vi "CPU Load Benchmark.vi"(8 "error in (no error)":errorcluster, 11 "SV B-M (Target) in":refnum<class "SV B-M (Target).lvclass">) -> (0 "error out":errorcluster, 3 "SV B-M (Target) out":refnum<class "SV B-M (Target).lvclass">)   [LabVIEW 2015, in "SV B-M (Target).lvclass"]
uses:
  SV B-M (Target).lvclass
  SV B-M (Target).lvclass/SV B-M (Target).ctl
  <vilib>/Analysis/baseanly.llb/Mean (DBL).vi
  <vilib>/nisyscfg/Close (Hardware).vi
  <vilib>/nisyscfg/Close (System).vi
  Command & Ack - Send Ack.vi
  <vilib>/nisyscfg/nisyscfg.lvlib
  <resource>/objmgr/nisysapi.rc
  <vilib>/Analysis/NI_AALBase.lvlib
panel:
  out "SV Data":variant[][](array[variant])
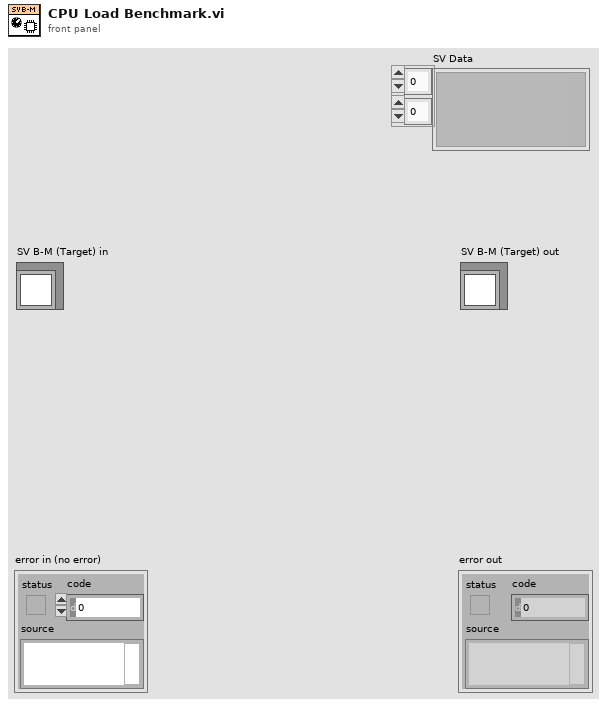
[diagram p1: front panel]
types:
  T1 = typedef "Variable Data Type.ctl" = enum16{"U8", "U16", "U32", "U64", "I8", "I16", "I32", "I64", "Single", "Double", "Boolean", "String"}
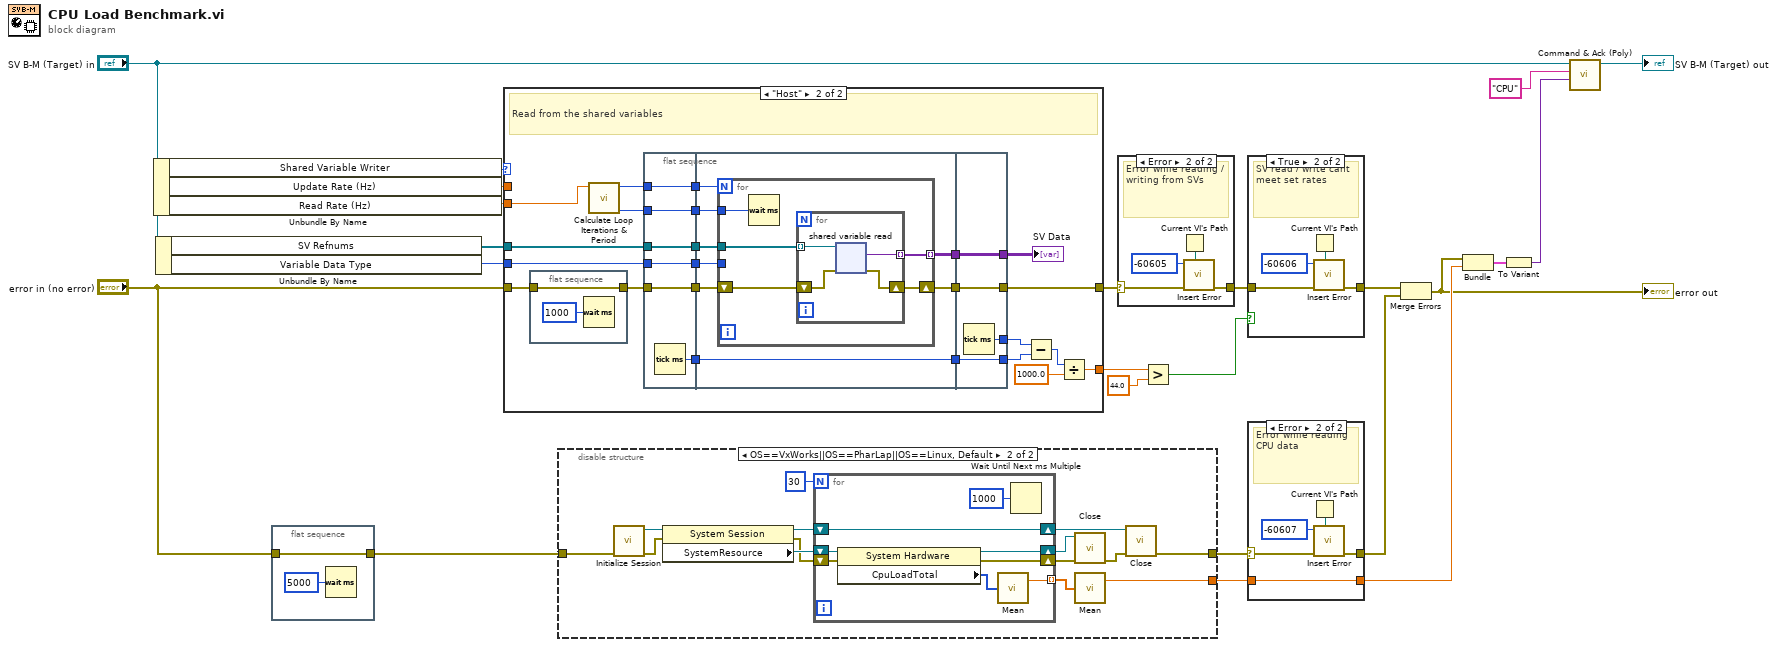
[diagram p0: block diagram]
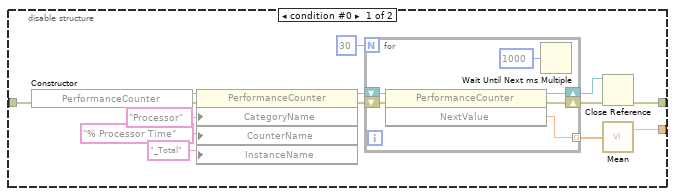
[diagram p3: hidden frame]
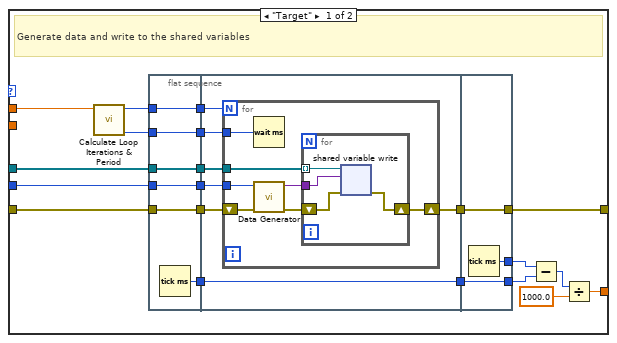
[diagram p6: hidden frame]
diagram:
  n1 = Unbundle By Name("SV B-M (Target) in") -> ("Shared Variable Writer"=w23:enum16{"Target", "Host"}, "Update Rate (Hz)"=w22:dbl, "Read Rate (Hz)"=w21:dbl)
  n2 = Unbundle By Name("SV B-M (Target) in") -> ("SV Refnums"=w20:refnum<k21>[], "Variable Data Type"=w19:T1)
  n3 = flat-sequence {
    tunnel: "error in (no error)" -> [w25]
    tunnel: [w25] -> w12
    frame #0 {
      n4 = Wait (ms)(milliseconds to wait=u32 5000) -> ()  [unwired: 1 out]
    }
  }
  n5 = case shown="\"Host\"" w23 {
    tunnel: w22 -> [w45 _]
    tunnel: w21 -> [_ w78]
    tunnel: w20 -> [w42 w93]
    tunnel: w19 -> [w41 w92]
    tunnel: "error in (no error)" -> [w36 w74]
    tunnel: [w27 w79] -> w15
    tunnel: [w26 w76] -> w18
    frame "Target" {
      # "Generate data and write to the shared variables"
      n6 = call "Calculate Loop Iterations & Period.vi"("Rate"=w45) -> ("Wait (ms)"=w43:u32, "# Iterations"=w44:i32)  [unwired: 9 in]
      n7 = flat-sequence {
        tunnel: w41 -> [w48]
        tunnel: w42 -> [w49]
        tunnel: w43 -> [w50]
        tunnel: w44 -> [w51]
        tunnel: [w51] -> w40
        tunnel: [w50] -> w39
        tunnel: [w49] -> w38
        tunnel: [w48] -> w37
        tunnel: w36 -> [w47]
        tunnel: [w47] -> w35
        tunnel: [w46] -> w34
        tunnel: w40 -> [w58]
        tunnel: w39 -> [w57]
        tunnel: w38 -> [w56]
        tunnel: w37 -> [w55]
        tunnel: w35 -> [w54]
        tunnel: w34 -> [w53]
        tunnel: [w53] -> w33
        tunnel: [w52] -> w32
        tunnel: [w72] -> w31
        tunnel: w33 -> [w72]
        tunnel: w32 -> [w70]
        tunnel: [w71] -> w30
        tunnel: [w70] -> w26
        frame #0 {
          n8 = Tick Count (ms)() -> (millisecond timer value=w46:u32)
        }
        frame #1 {
          n9 = for {
            N: w58 -> [_]
            tunnel: w57 -> [w65]
            tunnel: w56 -> [w62]
            tunnel: w55 -> [w64]
            shift-right: [w59] -> w52
            shift-left: w54 -> [w63]
            n10 = Wait (ms)(milliseconds to wait=w65) -> ()  [unwired: 1 out]
            n11 = call "Data Generator.vi"("error in (no error)"=w63, "Variable Data Type"=w64) -> ("error out"=w60:errorcluster, "Variant"=w61:variant)  [unwired: 8 in]
            n12 = for {
              tunnel: w62 -> [w69] mode=indexing
              tunnel: w61 -> [w67]
              shift-right: [w66] -> w59
              shift-left: w60 -> [w68]
              n13 = shared-variable-write(w69, w68, w67) -> (w66:errorcluster)  [unwired: 1 out]
            }
          }
        }
        frame #2 {
          n14 = Tick Count (ms)() -> (millisecond timer value=w71:u32)
        }
      }
      n15 = Subtract(x=w30, y=w31) -> (x-y=w29:u32)
      n16 = Divide(x=w29, y=1000.0) -> (x/y=w27:dbl)
    }
    frame "Host" {
      # "Read from the shared variables"
      n17 = flat-sequence {
        tunnel: w74 -> [w97]
        tunnel: [w97] -> w73
        frame #0 {
          n18 = Wait (ms)(milliseconds to wait=u32 1000) -> ()  [unwired: 1 out]
        }
      }
      n19 = call "Calculate Loop Iterations & Period.vi"("Rate"=w78) -> ("Wait (ms)"=w94:u32, "# Iterations"=w95:i32)  [unwired: 9 in]
      n20 = flat-sequence {
        tunnel: w92 -> [w100]
        tunnel: w93 -> [w101]
        tunnel: w94 -> [w102]
        tunnel: w95 -> [w103]
        tunnel: [w103] -> w91
        tunnel: [w102] -> w90
        tunnel: [w101] -> w89
        tunnel: [w100] -> w88
        tunnel: [w98] -> w87
        tunnel: [w99] -> w86
        tunnel: w73 -> [w98]
        tunnel: w91 -> [w111]
        tunnel: w90 -> [w110]
        tunnel: w89 -> [w109]
        tunnel: w88 -> [w108]
        tunnel: w87 -> [w107]
        tunnel: w86 -> [w106]
        tunnel: [w106] -> w85
        tunnel: [w105] -> w84
        tunnel: [w104] -> w77
        tunnel: [w124] -> w83
        tunnel: w85 -> [w124]
        tunnel: w84 -> [w121]
        tunnel: [w123] -> w82
        tunnel: [w122] -> w75
        tunnel: w77 -> [w122]
        tunnel: [w121] -> w76
        frame #0 {
          n21 = Tick Count (ms)() -> (millisecond timer value=w99:u32)
        }
        frame #1 {
          n22 = for {
            N: w111 -> [_]
            tunnel: w110 -> [w116]
            tunnel: w109 -> [w115]
            tunnel: w108 -> [_]
            shift-right: [w114] -> w105
            shift-left: w107 -> [w113]
            tunnel: [w112] -> w104 mode=indexing
            n23 = Wait (ms)(milliseconds to wait=w116) -> ()  [unwired: 1 out]
            n24 = for {
              tunnel: w115 -> [w120] mode=indexing
              shift-right: [w118] -> w114
              shift-left: w113 -> [w119]
              tunnel: [w117] -> w112 mode=indexing
              n25 = shared-variable-read(w120, w119) -> (w118:errorcluster, w117:variant)  [unwired: 2 out]
            }
          }
        }
        frame #2 {
          n26 = Tick Count (ms)() -> (millisecond timer value=w123:u32)
        }
      }
      n27 = Subtract(x=w82, y=w83) -> (x-y=w81:u32)
      n28 = Divide(x=w81, y=1000.0) -> (x/y=w79:dbl)
      "SV Data" <- w75
    }
  }
  n29 = disable-structure shown="OS==VxWorks||OS==PharLap||OS==Linux, Default" {
    disable-tunnel: w12 -> [w130 w158]
    disable-tunnel: [w125 w147] -> w11
    disable-tunnel: [w126 w146] -> w10
    frame condition #0 {
      n30 = constructor class="PerformanceCounter"(error in=w130) -> (reference out=w138:refnum<k24>, error out=w137:errorcluster)  [unwired: 2 in, 1 out]
      n31 = property class="PerformanceCounter"(reference=w138, error in=w137, "CategoryName"="Processor", "CounterName"="% Processor Time", "InstanceName"="_Total") -> (reference out=w136:refnum<k24>, error out=w135:errorcluster)
      n32 = for {
        N: 30 -> [_]
        shift-right: [w141] -> w128
        shift-left: w136 -> [w144]
        shift-right: [w140] -> w129
        shift-left: w135 -> [w143]
        tunnel: [w139] -> w127 mode=indexing
        n33 = invoke class="PerformanceCounter" method="NextValue"(reference=w144, error in=w143) -> (reference out=w141:refnum<k24>, error out=w140:errorcluster, "NextValue"=w139:sgl)  [unwired: 1 in]
        n34 = Wait Until Next ms Multiple(millisecond multiple=u32 1000 ("milliseconds to wait")) -> ()  [unwired: 1 out]
      }
      n35 = Close Reference(reference=w128, error in (no error)=w129) -> (error out=w125:errorcluster)
      n36 = call-poly <vilib>:"Mean.vi"("X"=w127) -> ("mean"=w126:dbl)  [unwired: 1 out]
    }
    frame condition #1 (active) {
      n37 = call <vilib>:"Initialize Session.vi"("error in (no error)"=w158) -> ("error out"=w156:errorcluster, "Session out"=w157:refnum<k21>)  [unwired: 9 in]
      n38 = property class="System Session"(reference=w157, error in=w156) -> (reference out=w154:refnum<k21>, error out=w153:errorcluster, "SystemResource"=w155:refnum<k20>)
      n39 = for {
        N: 30 -> [_]
        shift-right: [w163] -> w150
        shift-left: w155 -> [w165]
        shift-right: [w166] -> w148
        shift-left: w154 -> [w166]
        shift-right: [w162] -> w151
        shift-left: w153 -> [w164]
        tunnel: [w160] -> w152 mode=indexing
        n40 = property class="System Hardware"(reference=w165, error in=w164) -> (reference out=w163:refnum<k20>, error out=w162:errorcluster, "CpuLoadTotal"=w161:u32[])
        n41 = call-poly <vilib>:"Mean.vi"("X"=w161) -> ("mean"=w160:dbl)  [unwired: 1 out]
        n42 = Wait Until Next ms Multiple(millisecond multiple=u32 1000 ("milliseconds to wait")) -> ()  [unwired: 1 out]
      }
      n43 = call-poly <vilib>:"Close.vi"("error in (no error)"=w151, "Resource in"=w150) -> ("error out"=w149:errorcluster)  [unwired: 9 in]
      n44 = call-poly <vilib>:"Mean.vi"("X"=w152) -> ("mean"=w146:dbl)  [unwired: 1 out]
      n45 = call-poly <vilib>:"Close.vi"("error in (no error)"=w149, "Session in"=w148) -> ("error out"=w147:errorcluster)  [unwired: 9 in]
    }
  }
  n46 = case shown="Error" w18 {
    selector: w18 -> [w167 w169]
    tunnel: [w167 w168] -> w17
    frame No Error {
      # "No Error"
    }
    frame Error {
      # "Error while reading / writing from SVs"
      n47 = Current VI's Path() -> (path=w171:path)
      n48 = call "Insert Error.vi"("VI Path"=w171, "error in (no error)"=w169, "Error Code"=-60605) -> ("error out"=w168:errorcluster)  [unwired: 8 in]
    }
  }
  n49 = Greater?(x=w15, y=44.0) -> (0:w14:bool)
  n50 = case shown="True" w14 {
    tunnel: [w172 w174] -> w9
    tunnel: w17 -> [w172 w173]
    frame False {
      # "R/W rates met\nwithin 10%"
    }
    frame True {
      # "SV read / write cant\nmeet set rates"
      n51 = Current VI's Path() -> (path=w176:path)
      n52 = call "Insert Error.vi"("VI Path"=w176, "error in (no error)"=w173, "Error Code"=-60606) -> ("error out"=w174:errorcluster)  [unwired: 8 in]
    }
  }
  n53 = case shown="Error" w11 {
    selector: w11 -> [w178 w181]
    tunnel: [w178 w180] -> w8
    tunnel: [w177 w179] -> w7
    tunnel: w10 -> [w177 w179]
    frame No Error {
      # "No Error"
    }
    frame Error {
      # "Error while reading CPU data"
      n54 = Current VI's Path() -> (path=w183:path)
      n55 = call "Insert Error.vi"("VI Path"=w183, "error in (no error)"=w181, "Error Code"=-60607) -> ("error out"=w180:errorcluster)  [unwired: 8 in]
    }
  }
  n56 = Merge Errors(w9, w8) -> (w6:errorcluster)
  "error out" <- w6
  n57 = Bundle("error IO"=w6, "mean"=w7) -> (w3:cluster{"error IO":errorcluster, "mean":dbl})  [unwired: 1 in]
  n58 = To Variant(anything=w3) -> (Variant=w2:variant)
  n59 = call-poly "Command & Ack (Poly).vi"("Message Data"=w2, "Message"="CPU", "SV B-M (Target) In"="SV B-M (Target) in") -> ("SV B-M (Target) Out"=→"SV B-M (Target) out":refnum<class "SV B-M (Target).lvclass">)  [unwired: 6 in, 2 out]
